vi "Get Name.vi"(8 "error in (no error)":errorcluster, 11 "Blue Plugin in":refnum<class "Blue Plugin.lvclass">) -> (0 "error out":errorcluster, 2 "Get Name":string, 3 "Blue Plugin out":refnum<class "Blue Plugin.lvclass">)   [LabVIEW 2014, in "Blue Plugin.lvclass"]
uses:
  Blue Plugin.lvclass
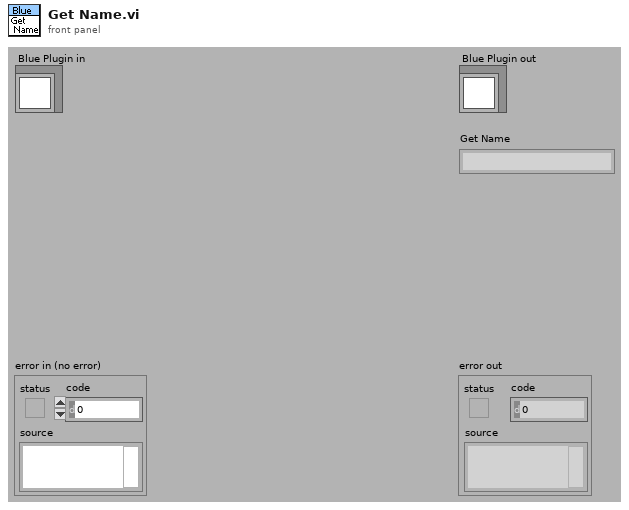
[diagram p1: front panel]
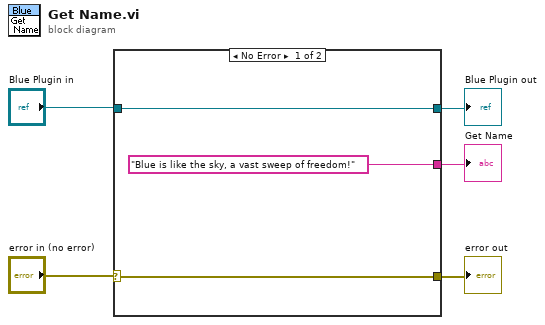
[diagram p0: block diagram]
diagram:
  n1 = case shown="No Error" "error in (no error)" {
    selector: "error in (no error)" -> [w8 w10]
    tunnel: [w8 w10] -> w4
    tunnel: ["Blue is like the sky, a vast sweep of freedom!" _] -> w3
    tunnel: [w6 w9] -> w2
    tunnel: "Blue Plugin in" -> [w6 w9]
    frame No Error {
    }
    frame Error {
    }
  }
  "error out" <- w4
  "Get Name" <- w3
  "Blue Plugin out" <- w2
